vi "UserFlatness.vi"(4 "Units":u16(ring)=1 items=["Hz", "MHz", "GHz"], 7 "cal file path (dialog if empty)":path=path "C:/RageATE/Automated Tests/Tetra WAM/DVT/Cal Files/SG1_CAL_073021-1514.csv", 8 "error in (no error)":errorcluster, 11 "Session In":refnum<visa-resource-name>="TCPIP0::169.254.70.100::inst0::INSTR") -> (0 "error out":errorcluster {"code" format="%.0x"}, 3 "Session Out":refnum<visa-resource-name>="TCPIP0::169.254.70.100::inst0::INSTR", 5 "success":bool)   [LabVIEW 2018, in "Agilent PSG MXG Series.lvlib"]
uses:
  Agilent PSG MXG Series.lvlib
  <vilib>/Utility/file.llb/Read Delimited Spreadsheet (string).vi
panel:
  out "Fstop":dbl
  out "Fstart":dbl
  out "Fpoints":i32
  out "Freq,Corr(dB)":dbl[][](array[numeric])
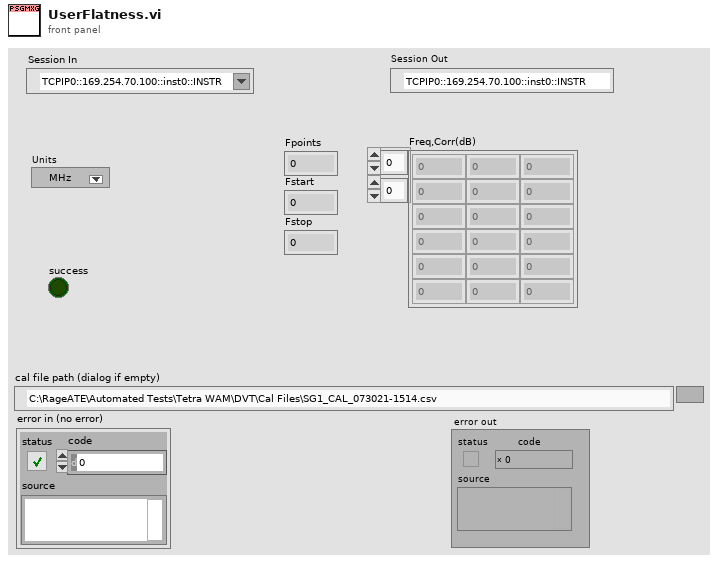
[diagram p1: front panel]
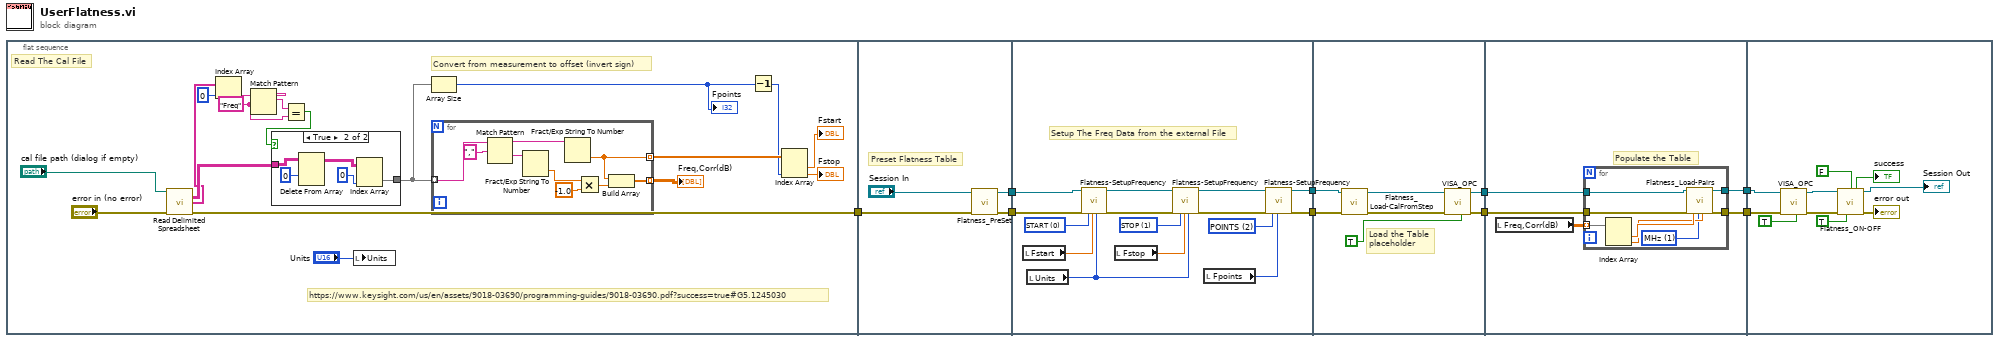
[diagram p0: block diagram]
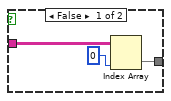
[diagram p2: hidden frame]
diagram:
  n1 = flat-sequence {
    tunnel: [w26] -> w9
    tunnel: w9 -> [w45]
    tunnel: [w48] -> w8
    tunnel: [w47] -> w7
    tunnel: w8 -> [w53]
    tunnel: w7 -> [w54]
    tunnel: [w51] -> w6
    tunnel: [w50] -> w5
    tunnel: w6 -> [w66]
    tunnel: w5 -> [w67]
    tunnel: [w65] -> w4
    tunnel: [w64] -> w3
    tunnel: w4 -> [w74]
    tunnel: w3 -> [w73]
    tunnel: [w72] -> w2
    tunnel: [w71] -> w1
    tunnel: w2 -> [w85]
    tunnel: w1 -> [w84]
    frame #0 {
      w11 = "Freq" ("regular expression")
      # "https://www.keysight.com/us/en/assets/9018-03690/programming-guides/9018-03690.pdf?success=true#G5.1245030"
      # "Convert from measurement to offset (invert sign)"
      # "Read The Cal File"
      n2 = call-poly <vilib>:"Read Delimited Spreadsheet.vi"("file path (dialog if empty)"="cal file path (dialog if empty)", "error in (no error)"="error in (no error)") -> ("all rows"=w16:string[][], "first row"=w14:string[], "error out"=w26:errorcluster)  [unwired: 8 in, 3 out]
      n3 = Index Array(array=w14, index=0 ("index (row)")) -> (element=w13:string)
      n4 = Match Pattern(string=w13, regular expression=w11) -> (match substring=w12:string)  [unwired: 1 in, 3 out]
      n5 = Equal?(x=w12, y=w11) -> (x = y?=w10:bool)
      n6 = case shown="True" w10 {
        tunnel: [w29 w34] -> w25
        tunnel: w16 -> [w28 w33]
        frame False {
          n7 = Index Array(array=w28, index (col)=0 ("disabled index (col)")) -> (element=w29:string[])  [unwired: 1 in]
        }
        frame True {
          n8 = Delete From Array(array=w33, index (row)=0) -> (array with subset deleted=w32:string[][])  [unwired: 2 in, 1 out]
          n9 = Index Array(array=w32, index (col)=0 ("disabled index (col)")) -> (element=w34:string[])  [unwired: 1 in]
        }
      }
      n10 = local write "Units"("Units") -> ()
      n11 = Array Size(array=w25) -> (size(s)=w22:i32)
      "Fpoints" <- w22
      n12 = for {
        tunnel: w25 -> [w44] mode=indexing
        tunnel: [w37] -> w24 mode=indexing
        tunnel: [w36] -> w23 mode=indexing
        n13 = Match Pattern(string=w44, regular expression=",") -> (before substring=w42:string, after substring=w41:string)  [unwired: 1 in, 2 out]
        n14 = Fract/Exp String To Number(string=w41) -> (number=w40:dbl)  [unwired: 3 in, 1 out]
        n15 = Fract/Exp String To Number(string=w42) -> (number=w36:dbl)  [unwired: 3 in, 1 out]
        n16 = Multiply(x=w40, y=-1.0) -> (x*y=w38:dbl)
        n17 = Build Array(w36, w38) -> (w37:dbl[])
      }
      "Freq,Corr(dB)" <- w24
      n18 = Decrement(x=w22) -> (x-1=w19:i32)
      n19 = Index Array(array=w23, index #2=w19) -> (element #1=→"Fstart":dbl, element #2=→"Fstop":dbl)  [unwired: 1 in]
    }
    frame #1 {
      # "Preset Flatness Table"
      n20 = call "Flatness_PreSet.vi"("error in"=w45, "Session In"="Session In") -> ("error out"=w48:errorcluster, "Session Out"=w47:refnum<visa-resource-name>)  [unwired: 7 in]
    }
    frame #2 {
      w56 = 2 items=["START", "STOP", "POINTS"] ("Select")
      w55 = 1 items=["START", "STOP", "POINTS"] ("Select")
      w52 = 0 items=["START", "STOP", "POINTS"] ("Select")
      # "Setup The Freq Data from the external File"
      n21 = local read "Fstart"() -> (w57:dbl)
      n22 = local read "Units"() -> (w49:u16)
      n23 = call "Flatness-SetupFrequency.vi"("Session In"=w54, "error in"=w53, "Select"=w52, "Freq/poin"=w57, "Units"=w49) -> ("Session Out"=w60:refnum<visa-resource-name>, "error out"=w59:errorcluster)  [unwired: 12 in, 1 out]
      n24 = local read "Fstop"() -> (w58:dbl)
      n25 = call "Flatness-SetupFrequency.vi"("Session In"=w60, "error in"=w59, "Select"=w55, "Freq/poin"=w58, "Units"=w49) -> ("Session Out"=w61:refnum<visa-resource-name>, "error out"=w62:errorcluster)  [unwired: 12 in, 1 out]
      n26 = local read "Fpoints"() -> (w63:i32)
      n27 = call "Flatness-SetupFrequency.vi"("Session In"=w61, "error in"=w62, "Select"=w56, "Freq/poin"=w63) -> ("Session Out"=w51:refnum<visa-resource-name>, "error out"=w50:errorcluster)  [unwired: 13 in, 1 out]
    }
    frame #3 {
      # "Load the Table\nplaceholder"
      n28 = call "Flatness_Load-CalFromStep.vi"("error in"=w67, "Session In"=w66) -> ("error out"=w70:errorcluster, "Session Out"=w69:refnum<visa-resource-name>)  [unwired: 8 in]
      n29 = call "VISA_OPC.vi"("OPC(T)"=TRUE ("OPC?(T)"), "error in"=w70, "Session In"=w69) -> ("error out"=w64:errorcluster, "Session Out"=w65:refnum<visa-resource-name>)  [unwired: 6 in, 1 out]
    }
    frame #4 {
      # "Populate the Table"
      n30 = local read "Freq,Corr(dB)"() -> (w75:dbl[][])
      n31 = for {
        tunnel: w75 -> [w83] mode=indexing
        tunnel: w74 -> [w80]
        tunnel: [w78] -> w72
        tunnel: [w77] -> w71
        tunnel: w73 -> [w76]
        w79 = u16 1 items=["Hz", "MHz", "GHz"] ("Freq Units")
        n32 = Index Array(array=w83) -> (element #1=w82:dbl, element #2=w81:dbl)  [unwired: 2 in]
        n33 = call "Flatness_Load-Pairs.vi"("Session In"=w80, "error in"=w76, "Freq"=w82, "Freq Units"=w79, "corr"=w81) -> ("Session Out"=w78:refnum<visa-resource-name>, "error out"=w77:errorcluster)  [unwired: 13 in]
      }
    }
    frame #5 {
      n34 = call "VISA_OPC.vi"("OPC(T)"=TRUE ("OPC?(T)"), "error in"=w84, "Session In"=w85) -> ("error out"=w91:errorcluster, "Session Out"=w90:refnum<visa-resource-name>)  [unwired: 6 in, 1 out]
      n35 = call "Flatness_ON-OFF.vi"("Session In"=w90, "RO(T)"=FALSE, "error in"=w91, "CORR ON(T)"=TRUE) -> ("success"=→"success":bool, "Session Out"=→"Session Out":refnum<visa-resource-name>, "error out"=→"error out":errorcluster)  [unwired: 9 in]
    }
  }
